vi "ContinueTestLogic.vi"(8 "error in (no error)":errorcluster, 11 "File IO Data in":T1 {"Test Information"."Run Count" min=0 step=1}) -> (0 "error out":errorcluster, 3 "File IO Data out":T1 {"Test Information"."Run Count" min=0 step=1})   [LabVIEW 2018, in "File IO.lvlib"]
uses:
  File IO.lvlib
  Private Controls/File IO Data.ctl
  <vilib>/Utility/NIReport.llb/NI_report.lvclass
  Controller (Host)/Public Controls/Test Information.ctl
  Controller (Host)/Public VIs/PreorPostSB.ctl
  Controller (Host)/Public Controls/APU Select.ctl
  Top Level/Shared Controls/Analyzed Data Sets.ctl
  Top Level/Shared Controls/All Data Cluster.ctl
  Top Level/Shared Controls/Acq Data.ctl
  Top Level/Shared Controls/APU Setup File.ctl
  Testing UI 1/Testing UI 1.lvlib
  Controller (Host)/Controller (Host).lvlib
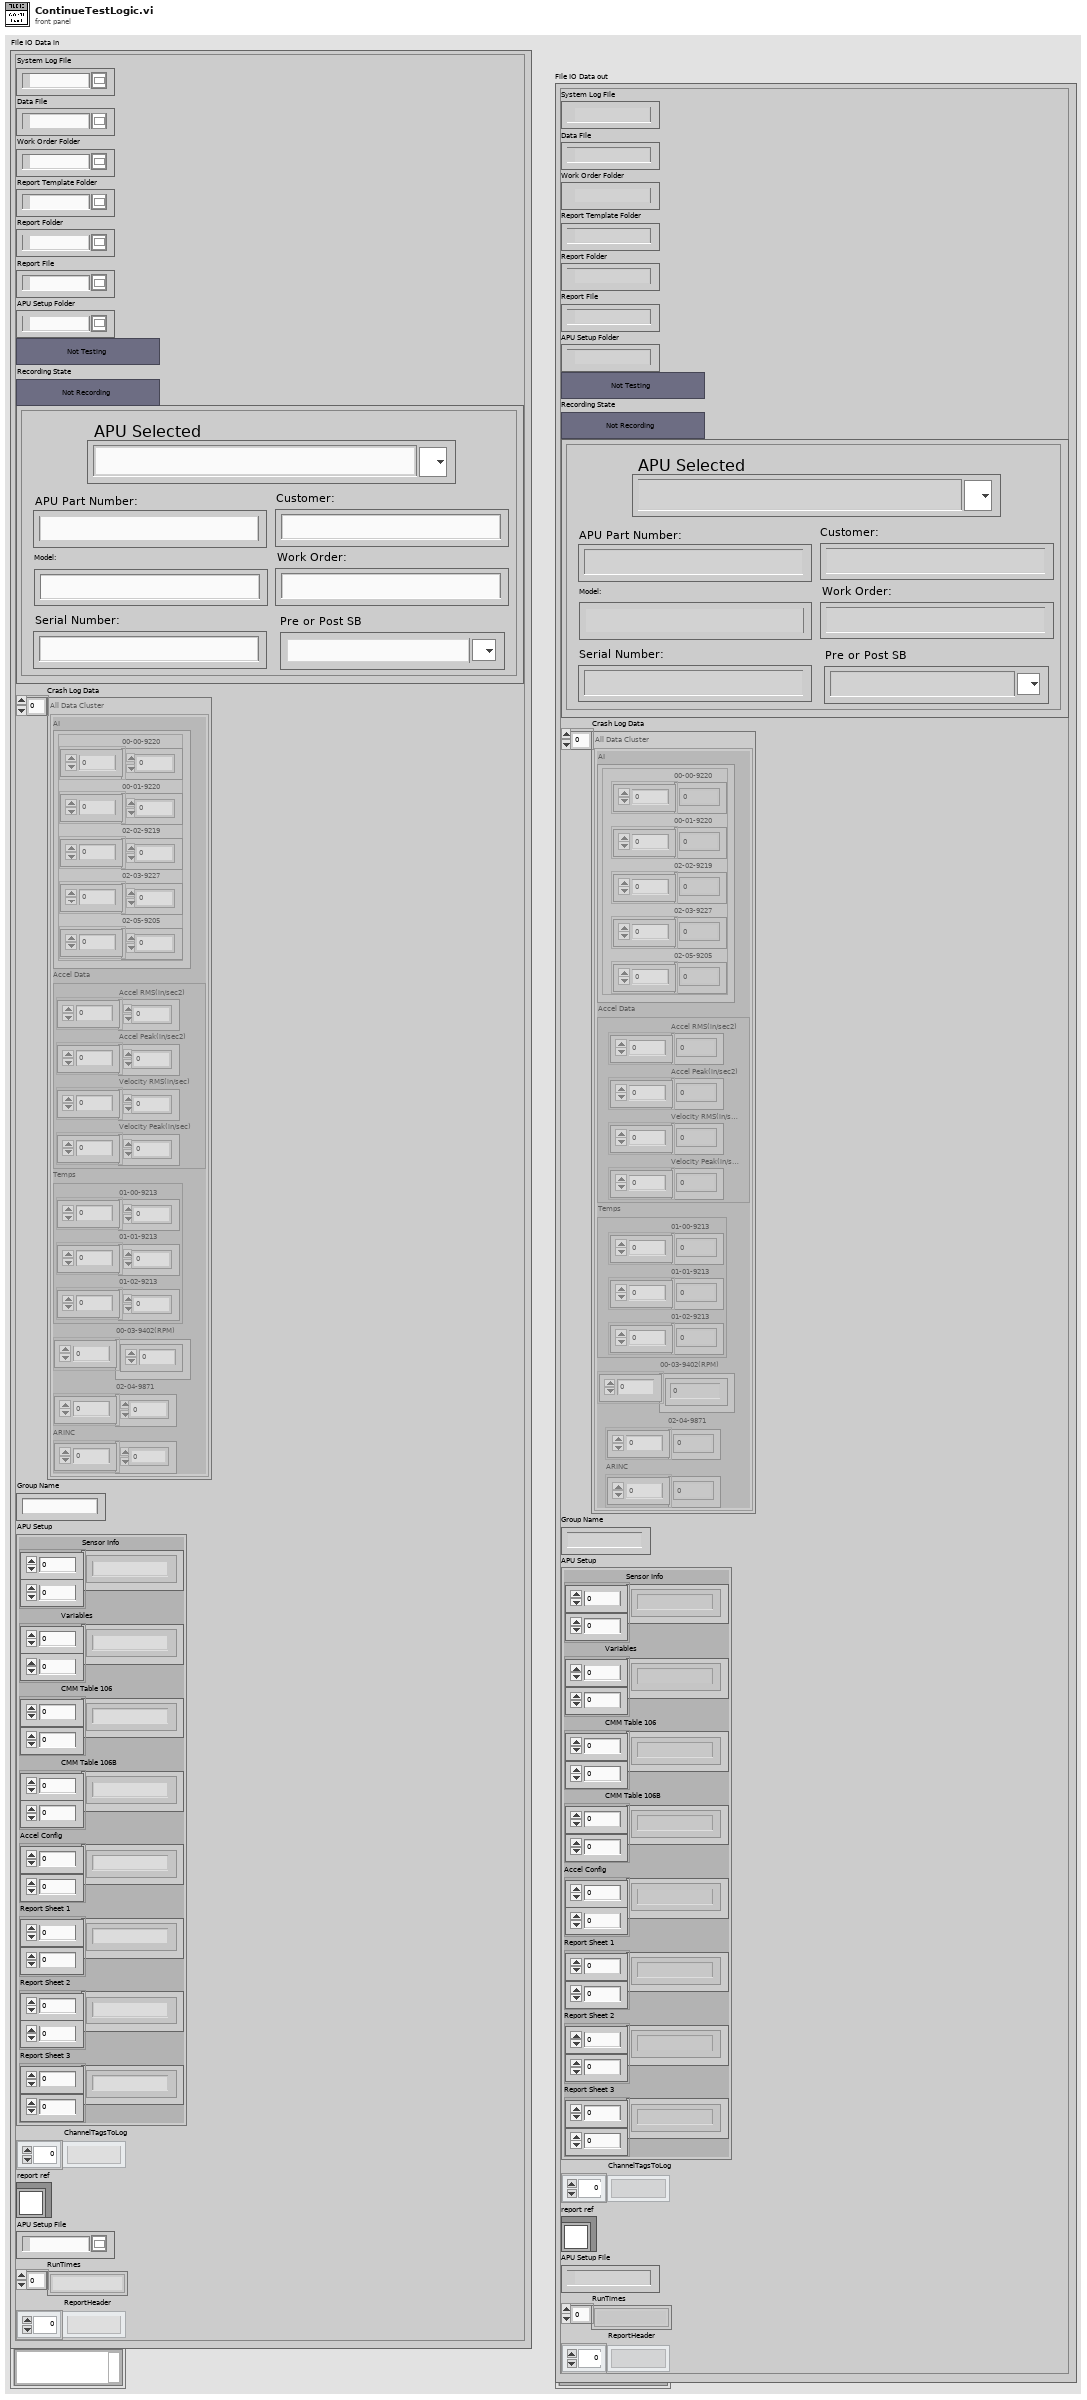
[diagram p1: front panel]
types:
  T1 = typedef "File IO.lvlib/File IO Data.ctl" = cluster{"System Log File":path, "Data File":path, "Work Order Folder":path, "Report Template Folder":path, "Report Folder":path, "Report File":path, "APU Setup Folder":path, "Testing State":bool, "Recording State":bool, "Test Information":T2, "Crash Log Data":T5, "Group Name":string, "APU Setup":T8, "ChannelTagsToLog":string[], "report ref":refnum<class "NI_report.lvclass">, "APU Setup File":path, "RunTimes":string[], "ReportHeader":string[]}
  T2 = typedef "Controller (Host).lvlib/Test Information.ctl" = cluster{"APU Part Number:":string, "Model:":string, "Serial Number:":string, "Customer:":string, "Work Order:":string, "Pre or Post SB":T3, "Run Count":i32, "APU Selected":T4}
  T3 = typedef "Controller (Host).lvlib/PreorPostSB.ctl" = string
  T4 = typedef "Controller (Host).lvlib/APU Select.ctl" = string
  T5 = typedef "Analyzed Data Sets.ctl" = T6[]
  T6 = typedef "All Data Cluster.ctl" = cluster{"AI":T7, "Accel Data":cluster{"Accel RMS(in/sec2)":dbl[], "Accel Peak(in/sec2)":dbl[], "Velocity RMS(in/sec)":dbl[], "Velocity Peak(in/sec)":dbl[]}, "Temps":cluster{"01-00-9213":dbl[], "01-01-9213":dbl[], "01-02-9213":dbl[]}, "00-03-9402(RPM)":dbl[], "02-04-9871":dbl[], "ARINC":sgl[]}
  T7 = typedef "Acq Data.ctl" = cluster{"00-00-9220":dbl[], "00-01-9220":dbl[], "02-02-9219":dbl[], "02-03-9227":dbl[], "02-05-9205":dbl[]}
  T8 = typedef "APU Setup File.ctl" = cluster{"Sensor Info":string[][], "Variables":string[][], "CMM Table 106":string[][], "CMM Table 106B ":string[][], "Accel Config":string[][], "Report Sheet 1":string[][], "Report Sheet 2":string[][], "Report Sheet 3":string[][]}
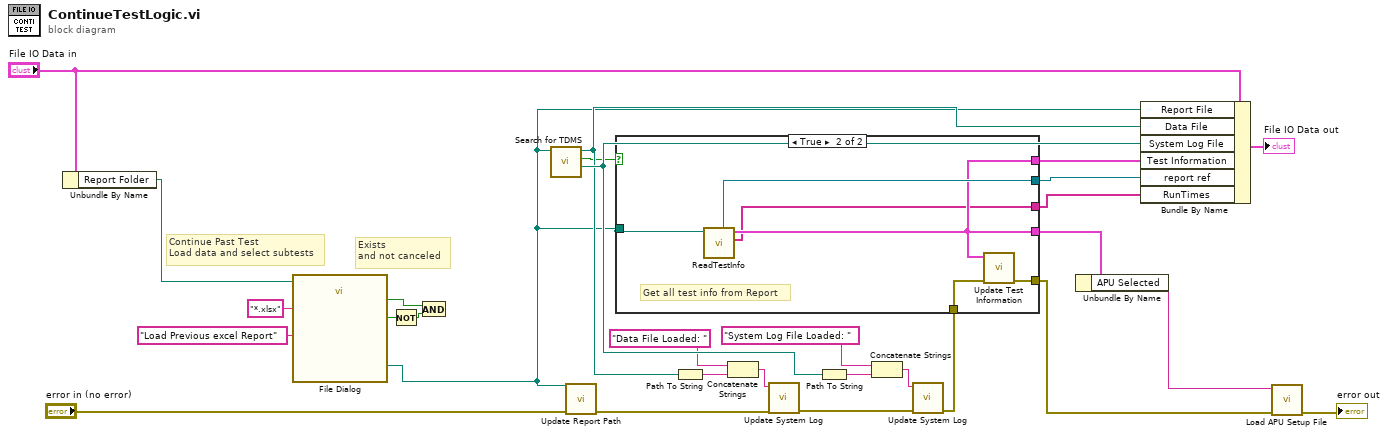
[diagram p0: block diagram]
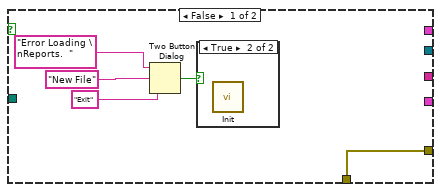
[diagram p2: hidden frame]
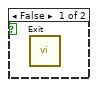
[diagram p3: hidden frame]
diagram:
  # "Exists\nand not canceled"
  # "Continue Past Test\nLoad data and select subtests"
  n1 = Unbundle By Name("File IO Data in") -> ("Report Folder"=w5:path)
  n2 = call "File Dialog"("start path"=w5, "prompt"="Load Previous excel Report", "pattern (all files)"="*.xlsx") -> ("selected path"=w4:path, "exists"=w8:bool, "cancelled"=w9:bool)  [unwired: 9 in, 1 out]
  n3 = Not(x=w9) -> (.not. x?=w10:bool)
  n4 = And(x=w8, y=w10) -> ()  [unwired: 1 out]
  n5 = call "Search for TDMS.vi"("Report Path"=w4) -> ("SystemLog"=w24:path, "Found?"=w13:bool, "Data File Path"=w18:path)  [unwired: 8 in]
  n6 = call "Update Report Path.vi"("error in (no error)"="error in (no error)", "Report Path"=w4) -> ("error out"=w15:errorcluster)  [unwired: 9 in]
  n7 = Path To String(path=w18) -> (string=w17:string)
  n8 = Concatenate Strings("Data File Loaded: " ("string"), w17) -> (w16:string)
  n9 = call "Update System Log.vi"("error in"=w15, "Message"=w16) -> ("error out"=w23:errorcluster)  [unwired: 9 in]
  n10 = Path To String(path=w24) -> (string=w21:string)
  n11 = Concatenate Strings("System Log File Loaded: " ("string"), w21) -> (w20:string)
  n12 = call "Update System Log.vi"("error in"=w23, "Message"=w20) -> ("error out"=w25:errorcluster)  [unwired: 9 in]
  n13 = case shown="True" w13 {
    tunnel: w4 -> [_ w40]
    tunnel: [_ w36] -> w14
    tunnel: w25 -> [w30 w39]
    tunnel: [w30 w38] -> w26
    tunnel: [_ w37] -> w28
    tunnel: [_ w36] -> w3
    tunnel: [_ w35] -> w1
    frame False {
      n14 = Two Button Dialog(message="Error Loading \nReports.  ", 1:"Exit" ("F button name (\"Cancel\")"), 2:"New File" ("T button name (\"OK\")")) -> (T button?=w31:bool)
      n15 = case shown="True" w31 {
        frame False {
          n16 = call "Exit.vi"() -> ()  [unwired: 11 in, 1 out]
        }
        frame True {
          n17 = call "Init.vi"() -> ()  [unwired: 11 in, 1 out]
        }
      }
    }
    frame True {
      # "Get all test info from Report"
      n18 = call "ReadTestInfo.vi"("Path"=w40) -> ("RunTimes"=w35:string[], "Test Information"=w36:T2, "report ref"=w37:refnum<class "NI_report.lvclass">)  [unwired: 7 in, 1 out]
      n19 = call "Update Test Information.vi"("error in"=w39, "Test Information"=w36) -> ("error out"=w38:errorcluster)  [unwired: 9 in]
    }
  }
  n20 = Unbundle By Name(w3) -> ("APU Selected"=w2:T4)
  n21 = Bundle By Name(cluster="File IO Data in", "Report File"=w4, "Data File"=w18, "System Log File"=w24, "Test Information"=w14, "report ref"=w28, "RunTimes"=w1) -> (→"File IO Data out":T1)
  n22 = call "Load APU Setup File.vi"("error in (no error)"=w26, "APU Select"=w2) -> ("error out"=→"error out":errorcluster)  [unwired: 9 in]
